vi "Format Client Request (Internal).vi"(8 "error in (no error)":errorcluster, 9 "params":variant, 10 "method":string) -> (0 "error out":errorcluster, 3 "JSON Tree out (JSON Object)":variant)   [LabVIEW 2015, in "JSONRPC Server.lvclass"]
uses:
  JSONRPC Server.lvclass
  <vilib>/NI/i3 JSON/JSON Generation/Create Value Files/Create Value - Object.vi
  <vilib>/NI/i3 JSON/JSON Generation/Add Object Parameter Files/Add Object Parameter - String.vi
  <vilib>/NI/i3 JSON/JSON Generation/Add Object Parameter Files/Add Object Parameter - Known Type.vi
  <vilib>/NI/i3 JSON/i3-json.lvlib
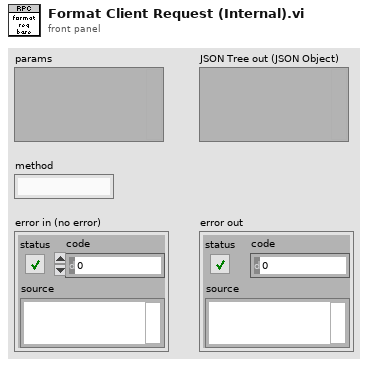
[diagram p1: front panel]
types:
  T1 = typedef "i3-json.lvlib/JSON Type.ctl" = enum8{"JSON Compatible", "JSON Array", "JSON Object", "JSON Null", "Double", "String", "Boolean", "Unknown"}
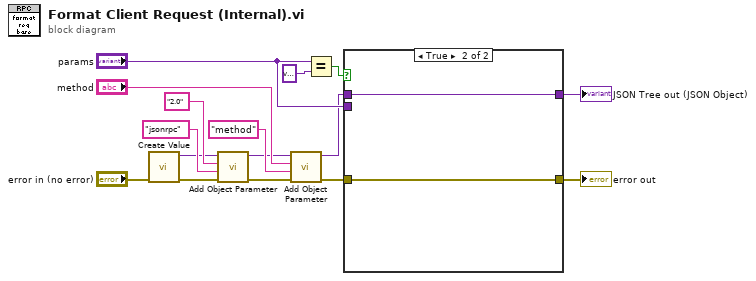
[diagram p0: block diagram]
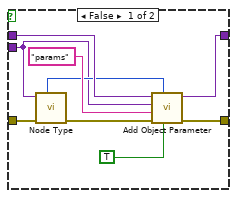
[diagram p2: hidden frame]
diagram:
  n1 = call-poly <vilib>:"Create Value.vi"("error in (no error)"="error in (no error)") -> ("error out"=w2:errorcluster, "JSON Tree"=w1:variant)  [unwired: 9 in]
  n2 = call-poly <vilib>:"Add Object Parameter.vi"("error in (no error)"=w2, "Name"="jsonrpc", "String"="2.0", "JSON Tree in (JSON Object)"=w1) -> ("error out"=w4:errorcluster, "JSON Tree out (JSON Object)"=w3:variant)  [unwired: 6 in]
  n3 = call-poly <vilib>:"Add Object Parameter.vi"("error in (no error)"=w4, "Name"="method", "String"="method", "JSON Tree in (JSON Object)"=w3) -> ("error out"=w5:errorcluster, "JSON Tree out (JSON Object)"=w6:variant)  [unwired: 6 in]
  n4 = Equal?(x="params", y=variant) -> (x = y?=w16:bool)
  n5 = case shown="True" w16 {
    tunnel: w5 -> [w25 w26]
    tunnel: w6 -> [w22 w27]
    tunnel: [w19 w27] -> w12
    tunnel: [w18 w26] -> w13
    tunnel: "params" -> [w17 _]
    frame False {
      n6 = call <vilib>:"Node Type.vi"("error in (no error)"=w25, "JSON Tree In"=w17) -> ("error out"=w24:errorcluster, "JSON Type"=w21:T1)  [unwired: 5 in, 3 out]
      n7 = call-poly <vilib>:"Add Object Parameter.vi"("Add Parameter as JSON Tree?"=TRUE, "JSON Type"=w21, "error in (no error)"=w24, "Name"="params", "Value"=w17, "JSON Tree in (JSON Object)"=w22) -> ("error out"=w18:errorcluster, "JSON Tree out (JSON Object)"=w19:variant)  [unwired: 4 in]
    }
    frame True {
    }
  }
  "error out" <- w13
  "JSON Tree out (JSON Object)" <- w12
